vi "Set IInstrument.vi"(8 "error in":errorcluster, 10 "IInstrument":refnum<class "IInstrument.lvclass">, 11 "NEO480 in":refnum<class "Virtual Thermometer.lvclass">) -> (0 "error out":errorcluster, 3 "NEO480 out":refnum<class "Virtual Thermometer.lvclass">)   [LabVIEW 2024, in "Virtual Thermometer.lvclass"]
uses:
  Virtual Thermometer.lvclass
  Interfaces/IInstrument/IInstrument.lvclass
  Interfaces/IRead Temperature/IRead Temperature.lvclass
  Virtual Thermometer.lvclass/Virtual Thermometer.ctl
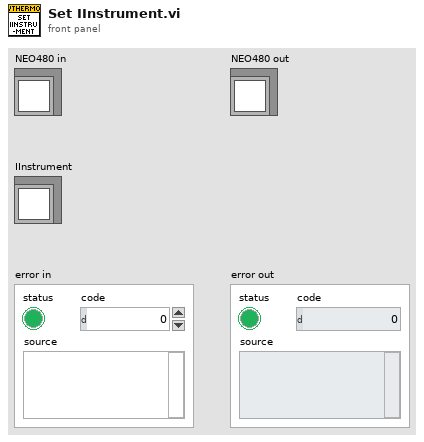
[diagram p1: front panel]
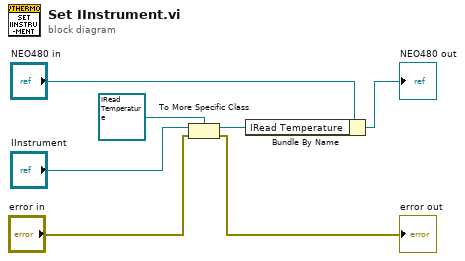
[diagram p0: block diagram]
diagram:
  n1 = To More Specific Class(target class=refnum<class "IRead Temperature.lvclass"> refnum ("IRead Temperature.lvclass"), reference="IInstrument", error in="error in") -> (specific class reference=w5:refnum<class "IRead Temperature.lvclass">, error out=→"error out":errorcluster)
  n2 = Bundle By Name(cluster="NEO480 in", "IRead Temperature"=w5) -> (→"NEO480 out":refnum<class "Virtual Thermometer.lvclass">)
